vi "Example1-Intro.vi"() -> ()   [LabVIEW 2020]
doc: "Example of value property and local variables usage."
uses:
  Ctrls/DataCluster.ctl
panel:
  in  "Calculate":bool
  in  "C":i8(knob) scale=0.0..10.0
  in  "B":i8(knob) scale=0.0..10.0
  in  "A":i8(knob) scale=0.0..10.0
  out "Data Chart":dbl(graph)
  in  "stop":bool
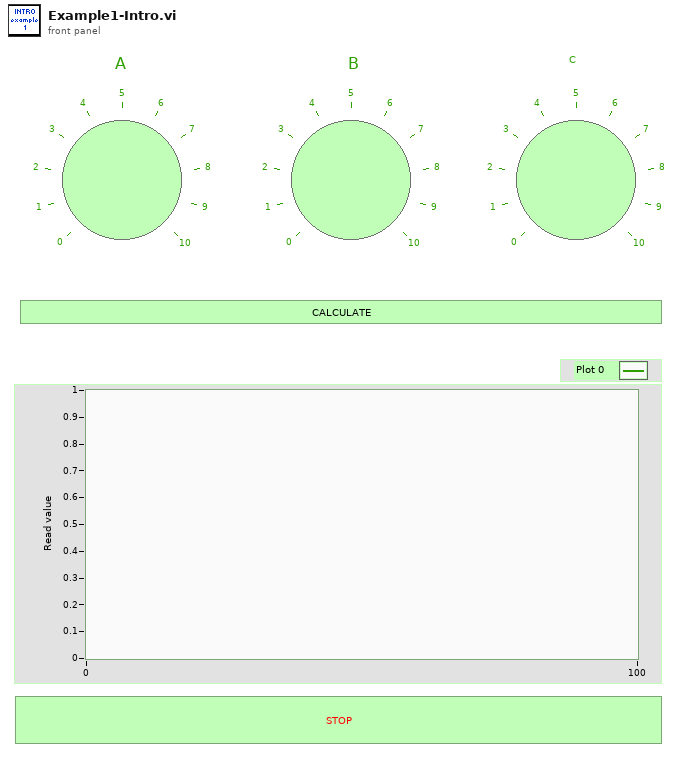
[diagram p1: front panel]
types:
  T1 = typedef "DataCluster.ctl" = cluster{"DataAndTime":timestamp, "Log message ":string, "Parameter 1":dbl}
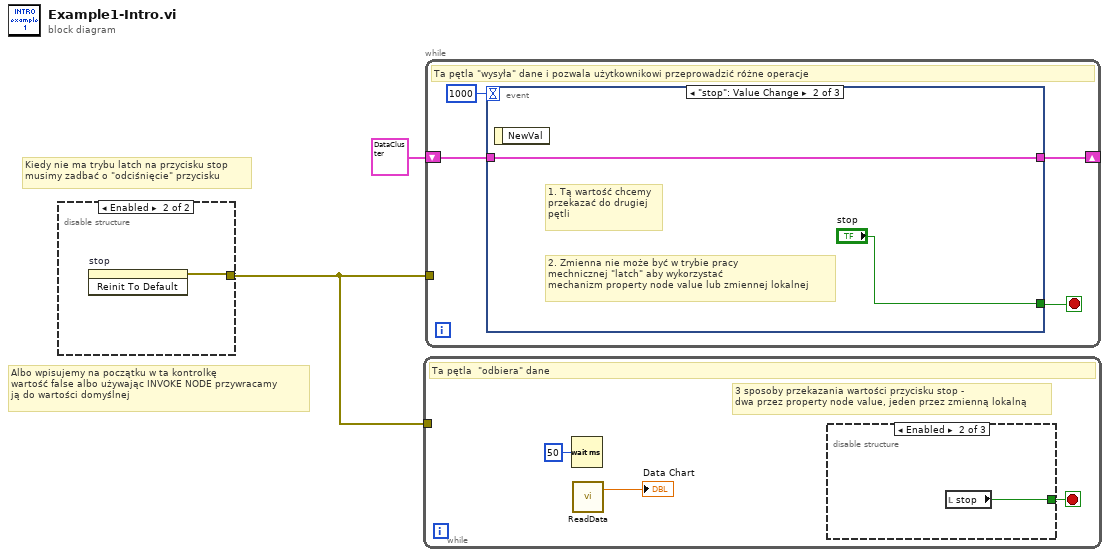
[diagram p0: block diagram]
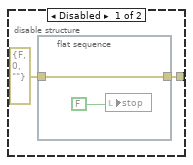
[diagram p2: hidden frame]
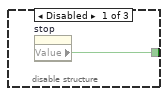
[diagram p3: hidden frame]
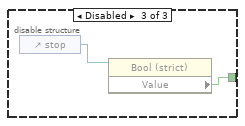
[diagram p4: hidden frame]
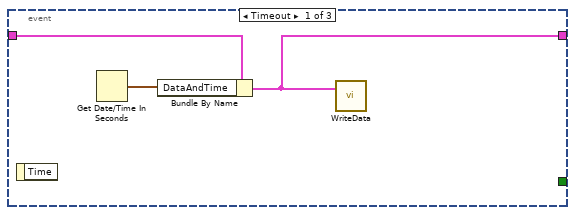
[diagram p5: hidden frame]
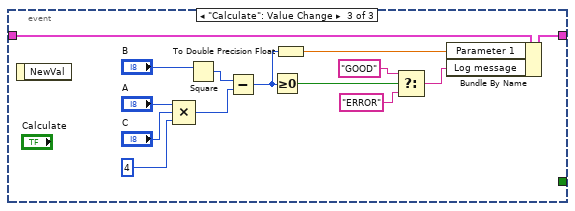
[diagram p6: hidden frame]
diagram:
  # "Albo wpisujemy na początku w ta kontrolkę \nwartość false albo używając INVOKE NODE przywracamy\nją do wartości domyślnej"
  # "Kiedy nie ma trybu latch na przycisku stop \nmusimy zadbać o \"odciśnięcie\" przycisku"
  n1 = disable-structure shown="Enabled" {
    disable-tunnel: [w4 w7] -> w1
    frame Disabled {
      n2 = flat-sequence {
        tunnel: errorcluster {"status"=FALSE, "code"=0, "source"=""} ("error out") -> [w6]
        tunnel: [w6] -> w4
        frame #0 {
          n3 = local write "stop"(FALSE ("Stop")) -> ()
        }
      }
    }
    frame Enabled {
      n4 = invoke on="stop" class="Bool (strict)" method="Reinit To Default"() -> (error out=w7:errorcluster)  [unwired: 3 in, 2 out]
    }
  }
  n5 = while {
    tunnel: w1 -> [_]
    stop <- w10 stop-if-true
    # "3 sposoby przekazania wartości przycisku stop -\ndwa przez property node value, jeden przez zmienną lokalną"
    # "Ta pętla  \"odbiera\" dane"
    n6 = Wait (ms)(milliseconds to wait=u32 50) -> ()  [unwired: 1 out]
    n7 = call "ReadData.vi"() -> ("number: 0 to 1"=→"Data Chart":dbl)  [unwired: 3 in]
    n8 = disable-structure shown="Enabled" {
      disable-tunnel: [w11 w12 w13] -> w10
      frame Disabled {
        n9 = property on="stop" class="Bool (strict)"() -> ("Value"=w11:bool)  [unwired: 2 in, 2 out]
      }
      frame Enabled {
        n10 = local read "stop"() -> (w12:bool)
      }
      frame Disabled {
        n11 = control-ref of="stop"() -> (w14:refnum<vi>)
        n12 = property class="Bool (strict)"(reference=w14) -> ("Value"=w13:bool)  [unwired: 1 in, 2 out]
      }
    }
  }
  n13 = while {
    shift-right: [w16] -> _
    shift-left: T1 {"DataAndTime"=timestamp(0 s since 1904-01-01), "Log message "="OK", "Parameter 1"=100.0} ("Data In") -> [w15]
    tunnel: w1 -> [_]
    stop <- w17 stop-if-true
    # "Ta pętla \"wysyła\" dane i pozwala użytkownikowi przeprowadzić różne operacje"
    n14 = event shown="[1] \"stop\": Value Change" {
      selector: _ -> [_ _ _]
      dyn-events: _ -> [_ _ _]
      timeout: 1000 ("Numeric") -> [_ _ _]
      tunnel: [_ "stop" _] -> w17
      tunnel: [w19 w22 w30] -> w16
      tunnel: w15 -> [w20 w22 w31]
      event Timeout {
        n15 = event-data() -> ()  [unwired: 1 in, 1 out]
        n16 = Get Date/Time In Seconds() -> (seconds since 1Jan1904=w21:timestamp)
        n17 = Bundle By Name(cluster=w20, "DataAndTime"=w21) -> (w19:T1)
        n18 = call "WriteData.vi"("Data In"=w19) -> ()  [unwired: 3 in]
      }
      event "stop": Value Change {
        # "2. Zmienna nie może być w trybie pracy\nmechnicznej \"latch\" aby wykorzystać \nmechanizm property node value lub zmiennej lokalnej"
        # "1. Tą wartość chcemy\nprzekazać do drugiej\npętli"
        n19 = event-data() -> ()  [unwired: 1 in, 1 out]
      }
      event "Calculate": Value Change {
        n20 = event-data() -> ()  [unwired: 1 in, 1 out]
        n21 = Compound Arithmetic op=MULTIPLY("A", "C", i8 4 ("value")) -> (w33:i8)
        n22 = Square(x="B") -> (x^2=w36:i8)
        n23 = Subtract(x=w36, y=w33) -> (x-y=w25:i8)
        n24 = Greater Or Equal To 0?(x=w25) -> (x >= 0?=w26:bool)
        n25 = To Double Precision Float(number=w25) -> (double precision float=w24:dbl)
        n26 = Select(t="GOOD", s=w26, f="ERROR") -> (s? t:f=w27:string)
        n27 = Bundle By Name(cluster=w31, "Parameter 1"=w24, "Log message"=w27) -> (w30:T1)
      }
    }
  }
